vi "Teardown.vi"(8 "error in (no error)":errorcluster, 11 "Dummy In":refnum<class "Dummy.lvclass">) -> (0 "error out":errorcluster, 3 "Dummy Out":refnum<class "Dummy.lvclass">)   [LabVIEW 2020, in "Dummy.lvclass"]
uses:
  Dummy.lvclass
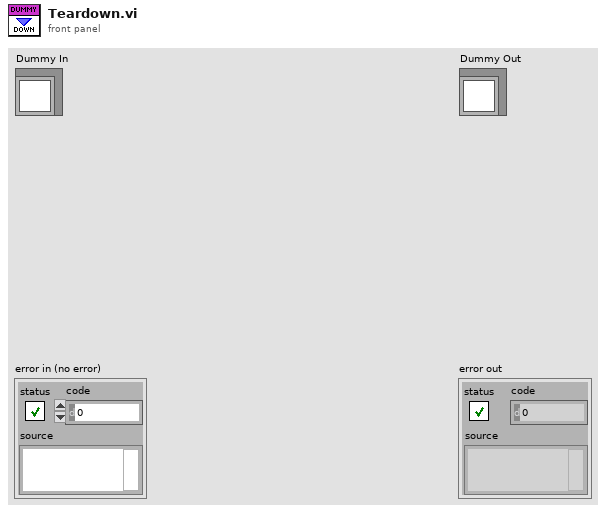
[diagram p1: front panel]
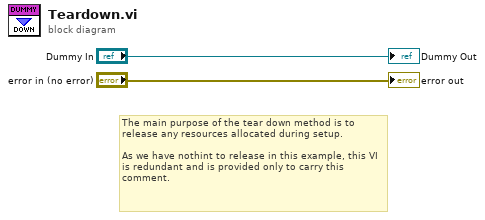
[diagram p0: block diagram]
diagram:
  # "The main purpose of the tear down method is to release any resources allocated during setup.\n \nAs we have nothint to release in this example, this VI is redundant and is provided only to carry this comment."
  "error out" <- "error in (no error)"
  "Dummy Out" <- "Dummy In"
